vi "Supervisor().vi"() -> (3 "Supervisor Out":refnum<class "Supervisor.lvclass">)   [LabVIEW 2014, in "Supervisor.lvclass"]
uses:
  Supervisor.lvclass
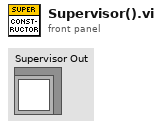
[diagram p1: front panel]
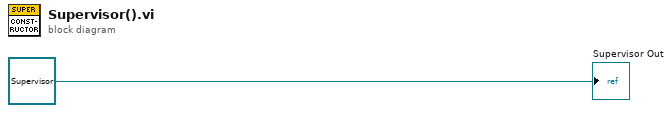
[diagram p0: block diagram]
diagram:
  "Supervisor Out" <- refnum<class "Supervisor.lvclass"> refnum ("Supervisor.lvclass")
